vi "Parse Response JSON.vi"(8 "error in (no error)":errorcluster, 10 "Response JSON":string, 11 "BatchResponse in":refnum<class "BatchResponse.lvclass">) -> (0 "error out":errorcluster, 3 "BatchResponse out":refnum<class "BatchResponse.lvclass">)   [LabVIEW 2020, in "obs-websocket.lvlib" / "BatchResponse.lvclass"]
uses:
  BatchResponse.lvclass
  BatchResponse.lvclass/BatchResponse.ctl
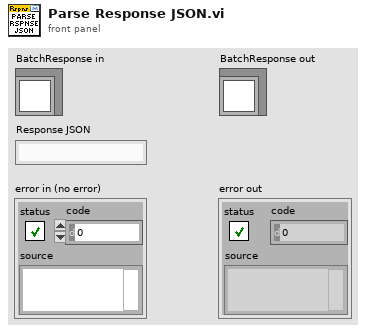
[diagram p1: front panel]
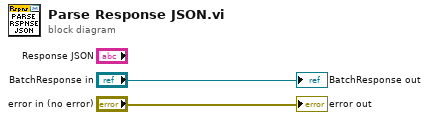
[diagram p0: block diagram]
diagram:
  "error out" <- "error in (no error)"
  "BatchResponse out" <- "BatchResponse in"
